vi "Heart Rate (SubVI).vi"(11 "Power Spectrum":dynamicdata(waveform)) -> (0 "Max Freq IR":dbl, 1 "Max Freq R":dbl, 2 "Array":dbl[](array[numeric]), 3 "Avg HR bpm":i32)   [LabVIEW 2021]
panel:
  in  "Period (s) in":dbl
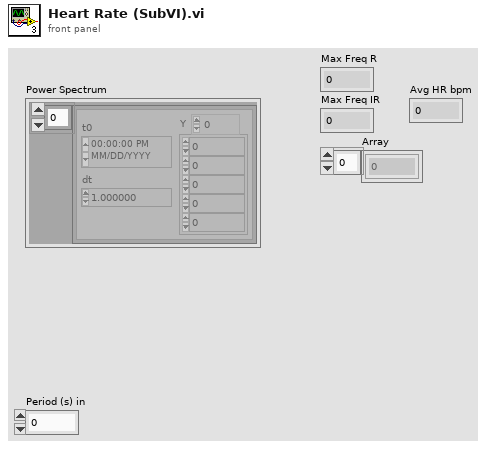
[diagram p1: front panel]
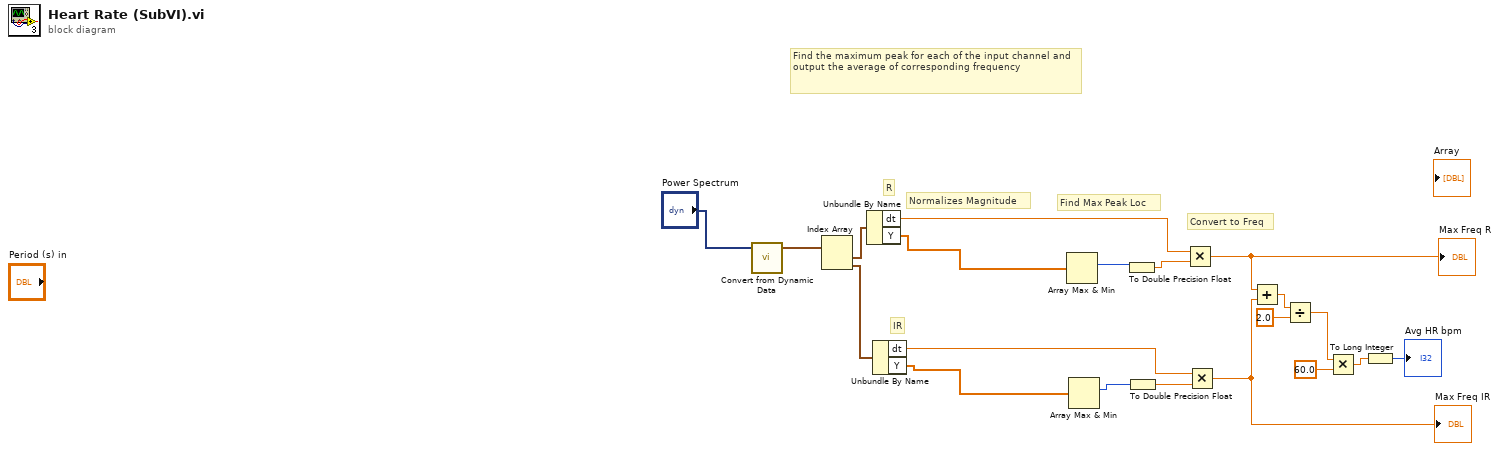
[diagram p0: block diagram]
diagram:
  # "Find the maximum peak for each of the input channel and output the average of corresponding frequency"
  # "Convert to Freq"
  # "Find Max Peak Loc"
  # "Normalizes Magnitude"
  # "IR"
  # "R"
  n1 = call "Convert from Dynamic Data"("Dynamic Data Type"="Power Spectrum") -> ("Array of Waveform"=w13:waveform(dbl)[])  [unwired: 3 in]
  n2 = Index Array(array=w13) -> (element #1=w12:waveform(dbl), element #2=w11:waveform(dbl))  [unwired: 2 in]
  n3 = Unbundle By Name(w12) -> ("dt"=w10:dbl, "Y"=w6:dbl[])
  n4 = Unbundle By Name(w11) -> ("dt"=w9:dbl, "Y"=w5:dbl[])
  n5 = Array Max & Min(array=w6) -> (max index (indices)=w4:i32)  [unwired: 3 out]
  n6 = Array Max & Min(array=w5) -> (max index (indices)=w2:i32)  [unwired: 3 out]
  n7 = To Double Precision Float(number=w4) -> (double precision float=w3:dbl)
  n8 = To Double Precision Float(number=w2) -> (double precision float=w1:dbl)
  n9 = Multiply(x=w10, y=w3) -> (x*y=w8:dbl)
  "Max Freq R" <- w8
  n10 = Multiply(x=w9, y=w1) -> (x*y=w7:dbl)
  "Max Freq IR" <- w7
  n11 = Add(x=w8, y=w7) -> (x+y=w17:dbl)
  n12 = Divide(x=w17, y=2.0) -> (x/y=w15:dbl)
  n13 = Multiply(x=w15, y=60.0) -> (x*y=w19:dbl)
  n14 = To Long Integer(number=w19) -> (32bit integer=→"Avg HR bpm":i32)
